vi "Get Voltage Scanner.vi"(8 "error in (no error)":errorcluster, 11 "Magna Power in":refnum<class "Magna Power.lvclass">) -> (0 "error out":errorcluster, 2 "Default Scanner out":refnum<class "Scanner.lvclass">)   [LabVIEW 2012, in "Magna Power.lvclass"]
uses:
  Magna Power.lvclass
  Scanners/Scanner/Scanner.lvclass
  Scanners/Magna Voltage Scan/Magna Voltage Scan.lvclass
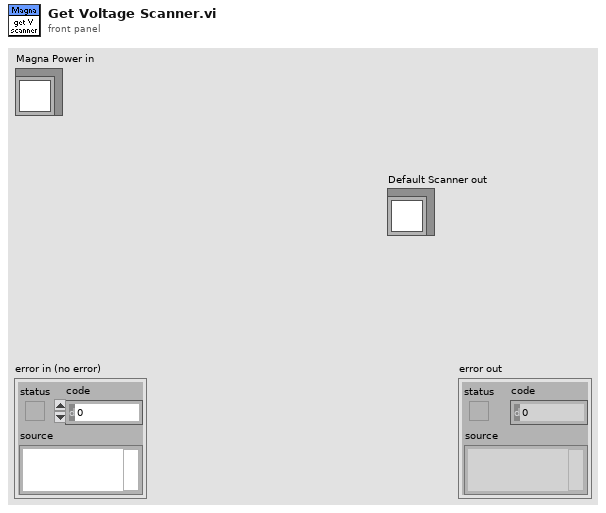
[diagram p1: front panel]
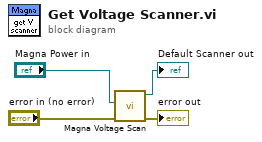
[diagram p0: block diagram]
diagram:
  n1 = call "Magna Voltage Scan.vi"("error in (no error)"="error in (no error)", "Magna Power.lvclass"="Magna Power in") -> ("error out"=→"error out":errorcluster, "Magna Voltage Scan.lvclass 2"=→"Default Scanner out":refnum<class "Magna Voltage Scan.lvclass">)  [unwired: 8 in]
